vi "Servo_Pan_Tilt.vi"(0 "Tilt_Servo_Position":dbl, 1 "Pan_Servo_Position":dbl, 2 "Smooth?":bool=TRUE, 3 "Tilt_Servo_Name":string="Tilt_Servo", 4 "Pan_Servo_Name":string="Pan_Servo") -> ()   [LabVIEW 2013]
uses:
  <vilib>/addons/control/pid/pid.llb/PID Control Input Filter (DBL).vi
  <vilib>/addons/control/pid/NI_PID_pid.lvlib
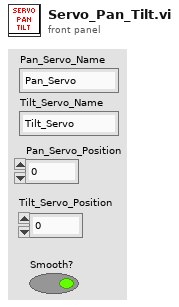
[diagram p1: front panel]
types:
  T1 = typedef "WPI_ServoDeviceRef.ctl" = cluster{"DeviceStatus":errorcluster, "Digital Module":T2, "PWM Channel":T3, "DeadBand":T4}
  T2 = typedef "FPGA_TypedefDigitalModule.ctl" = enum16{"Digital Module 1", "Digital Module 2"}
  T3 = typedef "FPGA_DIOPWMChannel.ctl" = enum8{"PWM 1", "PWM 2", "PWM 3", "PWM 4", "PWM 5", "PWM 6", "PWM 7", "PWM 8", "PWM 9", "PWM 10", "Invalid"}
  T4 = typedef "WPI_PWMDeadband.ctl" = cluster{"Name":string, "maxPositivePwm":i32, "minPositivePwm":i32, "centerPwm":i32, "maxNegativePwm":i32, "minNegativePwm":i32, "angularRange":u16}
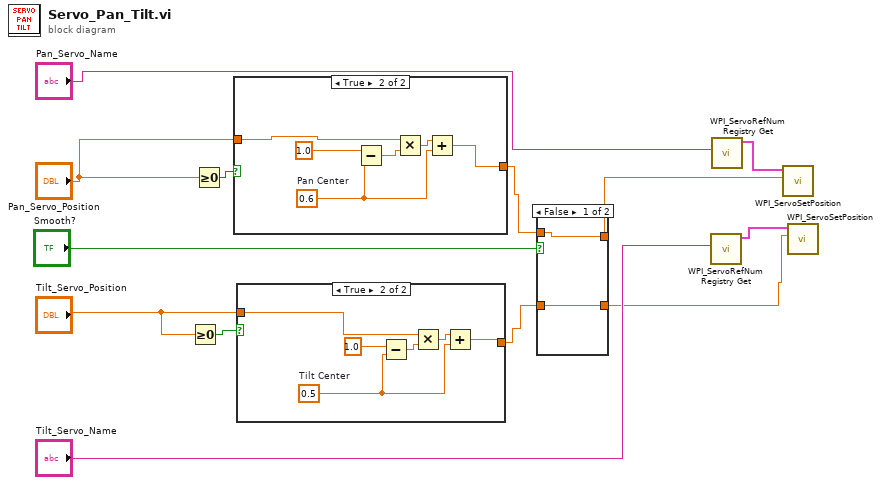
[diagram p0: block diagram]
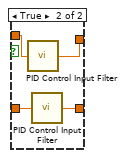
[diagram p2: hidden frame]
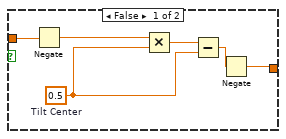
[diagram p3: hidden frame]
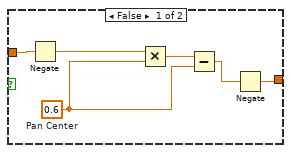
[diagram p4: hidden frame]
diagram:
  n1 = Greater Or Equal To 0?(x="Tilt_Servo_Position") -> (x >= 0?=w12:bool)
  n2 = Greater Or Equal To 0?(x="Pan_Servo_Position") -> (x >= 0?=w13:bool)
  n3 = case shown="True" w13 {
    tunnel: [w15 w20] -> w4
    tunnel: "Pan_Servo_Position" -> [w18 w24]
    frame False {
      w16 = 0.6  # Pan Center
      n4 = Negate(x=w18) -> (-x=w17:dbl)
      n5 = Multiply(x=w17, y=w16) -> (x*y=w19:dbl)
      n6 = Subtract(x=w19, y=w16) -> (x-y=w14:dbl)
      n7 = Negate(x=w14) -> (-x=w15:dbl)
    }
    frame True {
      w21 = 0.6  # Pan Center
      n8 = Subtract(x=1.0, y=w21) -> (x-y=w23:dbl)
      n9 = Multiply(x=w24, y=w23) -> (x*y=w25:dbl)
      n10 = Add(x=w25, y=w21) -> (x+y=w20:dbl)
    }
  }
  n11 = case shown="True" w12 {
    tunnel: [w26 w33] -> w3
    tunnel: "Tilt_Servo_Position" -> [w27 w32]
    frame False {
      w29 = 0.5  # Tilt Center
      n12 = Negate(x=w27) -> (-x=w30:dbl)
      n13 = Multiply(x=w30, y=w29) -> (x*y=w31:dbl)
      n14 = Subtract(x=w31, y=w29) -> (x-y=w28:dbl)
      n15 = Negate(x=w28) -> (-x=w26:dbl)
    }
    frame True {
      w34 = 0.5  # Tilt Center
      n16 = Subtract(x=1.0, y=w34) -> (x-y=w36:dbl)
      n17 = Multiply(x=w32, y=w36) -> (x*y=w37:dbl)
      n18 = Add(x=w37, y=w34) -> (x+y=w33:dbl)
    }
  }
  n19 = case shown="False" "Smooth?" {
    tunnel: w4 -> [w39 w43]
    tunnel: w3 -> [w38 w42]
    tunnel: [w38 w41] -> w2
    tunnel: [w39 w40] -> w1
    frame False {
    }
    frame True {
      n20 = call-poly <vilib>:"PID Control Input Filter.vi"("input"=w43) -> ("output"=w40:dbl)  [unwired: 1 in, 3 out]
      n21 = call-poly <vilib>:"PID Control Input Filter.vi"("input"=w42) -> ("output"=w41:dbl)  [unwired: 1 in, 3 out]
    }
  }
  n22 = call <vilib>:"WPI_ServoRefNum Registry Get.vi"("refnum name"="Tilt_Servo_Name") -> ("ServoDeviceRef"=w8:T1)  [unwired: 9 in, 1 out]
  n23 = call <vilib>:"WPI_ServoRefNum Registry Get.vi"("refnum name"="Pan_Servo_Name") -> ("ServoDeviceRef"=w9:T1)  [unwired: 9 in, 1 out]
  n24 = call <vilib>:"WPI_ServoSetPosition.vi"("Position"=w1, "ServoDeviceRef"=w9) -> ()  [unwired: 8 in, 2 out]
  n25 = call <vilib>:"WPI_ServoSetPosition.vi"("Position"=w2, "ServoDeviceRef"=w8) -> ()  [unwired: 8 in, 2 out]
